vi "onConnection.vi"(8 "error in (no error)":errorcluster, 11 "Connection.NetworkStream in":refnum<class "Connection.NetworkStream.lvclass">) -> (0 "error out":errorcluster, 3 "Connection.NetworkStream out":refnum<class "Connection.NetworkStream.lvclass">)   [LabVIEW 2013]
uses:
  Connection.NetworkStream.lvclass
  Connection/Connection.lvclass
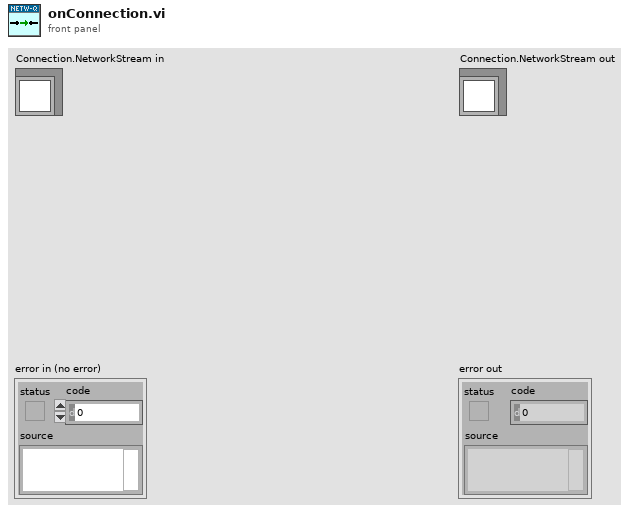
[diagram p1: front panel]
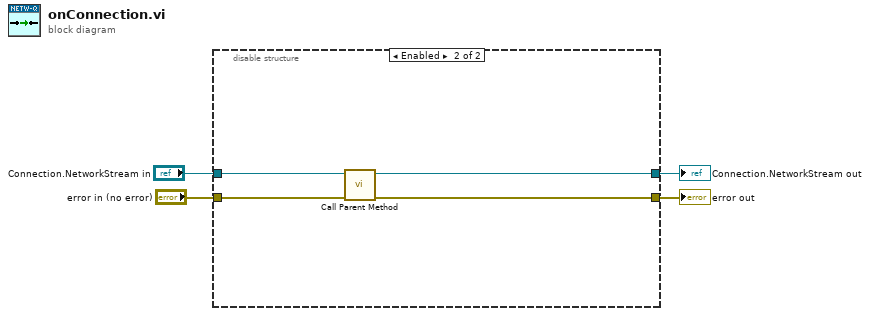
[diagram p0: block diagram]
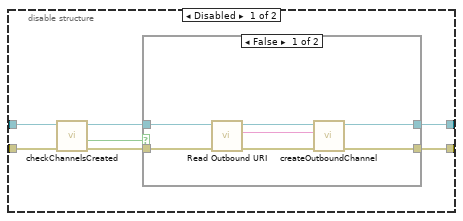
[diagram p2: hidden frame]
diagram:
  n1 = disable-structure shown="Enabled" {
    disable-tunnel: "Connection.NetworkStream in" -> [w8 w23]
    disable-tunnel: "error in (no error)" -> [w7 w22]
    disable-tunnel: [w6 w20] -> w2
    disable-tunnel: [w5 w21] -> w1
    frame Disabled {
      n2 = call-dynamic "checkChannelsCreated.vi"("error in (no error)"=w7, "Connection.NetworkStream in"=w8) -> ("error out"=w10:errorcluster, "outbound created"=w11:bool, "Connection.NetworkStream out"=w9:refnum<class "Connection.NetworkStream.lvclass">)  [unwired: 6 in, 1 out]
      n3 = case shown="False" w11 {
        tunnel: w10 -> [w12 w18]
        tunnel: [w16 w18] -> w5
        tunnel: w9 -> [w14 w19]
        tunnel: [w17 w19] -> w6
        frame False {
          n4 = call "Read Outbound URI.vi"("Connection in"=w14) -> ("Outbound URI"=w15:string, "Connection out"=w13:refnum<class "Connection.NetworkStream.lvclass">)  [unwired: 9 in]
          n5 = call-dynamic "createOutboundChannel.vi"("error in (no error)"=w12, "redirect"=w15, "Connection.NetworkStream in"=w13) -> ("error out"=w16:errorcluster, "Connection.NetworkStream out"=w17:refnum<class "Connection.NetworkStream.lvclass">)  [unwired: 7 in]
        }
        frame True {
        }
      }
    }
    frame Enabled {
      n6 = call-parent "Call Parent Method"("error in (no error)"=w22, "Connection in"=w23) -> ("error out"=w21:errorcluster, "Connection out"=w20:refnum<class "Connection.NetworkStream.lvclass">)  [unwired: 8 in]
    }
  }
  "error out" <- w1
  "Connection.NetworkStream out" <- w2
